vi "ds get serial number by index.vi"(10 "serial_number":u32, 11 "docking_station_index":i32) -> (2 "serial_number out":u32, 3 "function return":i32)   [LabVIEW 2019, in "apdm.lvlib"]
doc: "APDM_EXPORT int apdm_ds_get_serial_number_by_index(const int docking_station_index, uint32_t *serial_number);"
uses:
  apdm.lvlib
  Lee Lab/CP FES Walking 2018/Code/Working/LabVIEW/apdm.dll
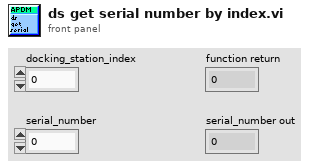
[diagram p1: front panel]
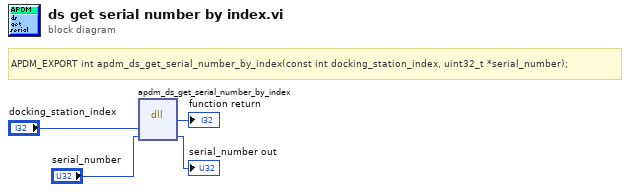
[diagram p0: block diagram]
diagram:
  # "APDM_EXPORT int apdm_ds_get_serial_number_by_index(const int docking_station_index, uint32_t *serial_number);"
  n1 = dll-call lib="C:/Users/jfalesi/Dropbox/Lee Lab/CP FES Walking 2018/Code/Working/LabVIEW/apdm.*" fn="apdm_ds_get_serial_number_by_index"("docking_station_index"="docking_station_index", "serial_number"="serial_number") -> (→"function return":i32, "serial_number"=→"serial_number out":u32)  [unwired: 4 in, 2 out]
